vi "Einheiten in Tabellenspalten Strings.vi"(8 "Fehler (Eingang, kein Fehler)":errorcluster, 10 "Spalten Titel mit Einheiten in":string[](array[string]), 11 "Einheit in":string) -> (0 "Fehler (Ausgang)":errorcluster, 2 "Spalten Titel mit Einheiten out":string[](array[string]), 3 "Einheit out":string)   [LabVIEW 2020, in "Linearisierung v2.lvlib"]
uses:
  Linearisierung v2.lvlib
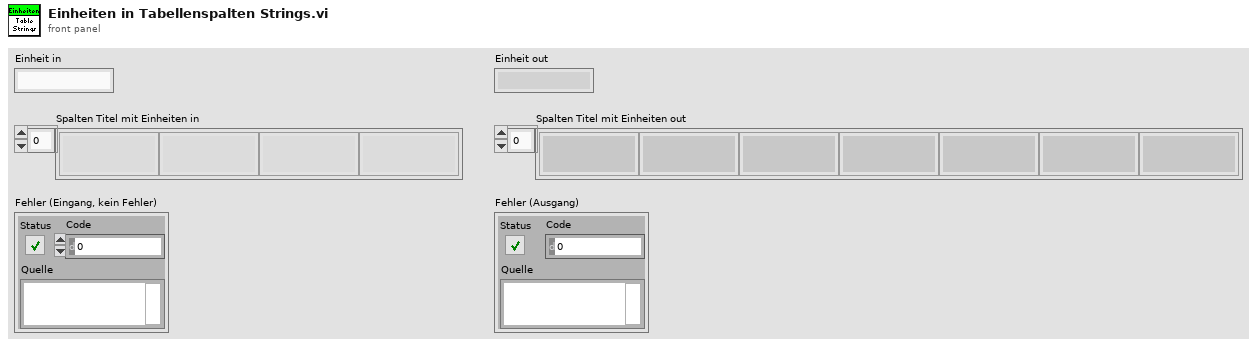
[diagram p1: front panel]
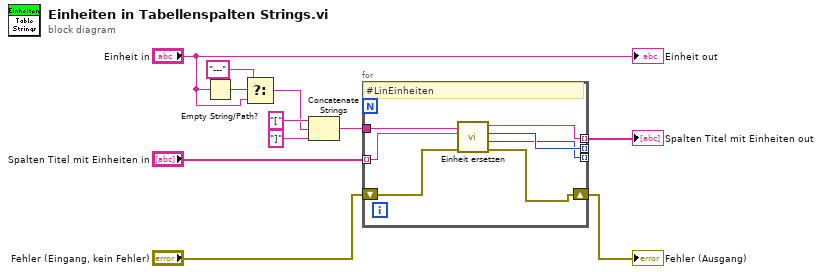
[diagram p0: block diagram]
diagram:
  n1 = Empty String/Path?(string/path="Einheit in") -> (empty?=w4:bool)
  n2 = Select(t="---", s=w4, f="Einheit in") -> (s? t:f=w1:string)
  n3 = Concatenate Strings("[" ("String"), w1, "]" ("String")) -> (w5:string)
  n4 = for {
    tunnel: "Spalten Titel mit Einheiten in" -> [w18] mode=indexing
    tunnel: w5 -> [w14]
    shift-right: [w16] -> w10
    shift-left: "Fehler (Eingang, kein Fehler)" -> [w17]
    tunnel: [w15] -> w9 mode=indexing
    tunnel: [w13] -> _ mode=indexing
    tunnel: [w12] -> _ mode=indexing
    # "#LinEinheiten"
    n5 = call "Einheit ersetzen.vi"("Fehler (Eingang, kein Fehler)"=w17, "Spaltentiitel"=w18, "Einheit"=w14) -> ("Fehler (Ausgang)"=w16:errorcluster, "offset past replacement"=w12:i32, "number of replacements"=w13:i32, "result string"=w15:string)  [unwired: 5 in]
  }
  "Fehler (Ausgang)" <- w10
  "Spalten Titel mit Einheiten out" <- w9
  "Einheit out" <- "Einheit in"
